vi "CloseDS.vi"(1 "DataSocket Refnum":refnum<k13>) -> (0 "error out":errorcluster)   [LabVIEW 2010]
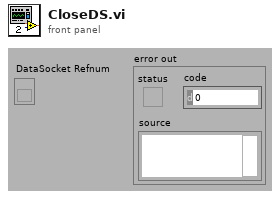
[diagram p1: front panel]
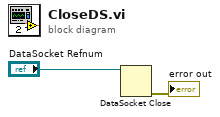
[diagram p0: block diagram]
diagram:
  n1 = DataSocket Close(11:"DataSocket Refnum") -> (0:→"error out":errorcluster)  [unwired: 1 in, 2 out]
